vi "Get Argument Info From back Term.vi"(11 "Terminal in":refnum<vi>) -> (3 "Array":T1[](array[typedef]))   [LabVIEW 2020, in "CSM-Helper.lvclass"]
uses:
  CSM-Helper.lvclass
  Typedef/Def-Argument Info.ctl
  CSM-Helper.lvclass/CSM-Helper.ctl
  <userlib>/_NEVSTOP/Communicable State Machine(CSM)/Communicable State Machine.lvlib
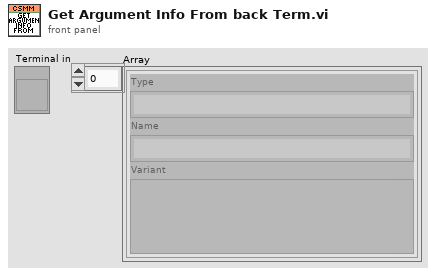
[diagram p1: front panel]
types:
  T1 = typedef "CSM-Helper.lvclass/Def-Argument Info.ctl" = cluster{"Type":string, "Name":string, "Variant":variant}
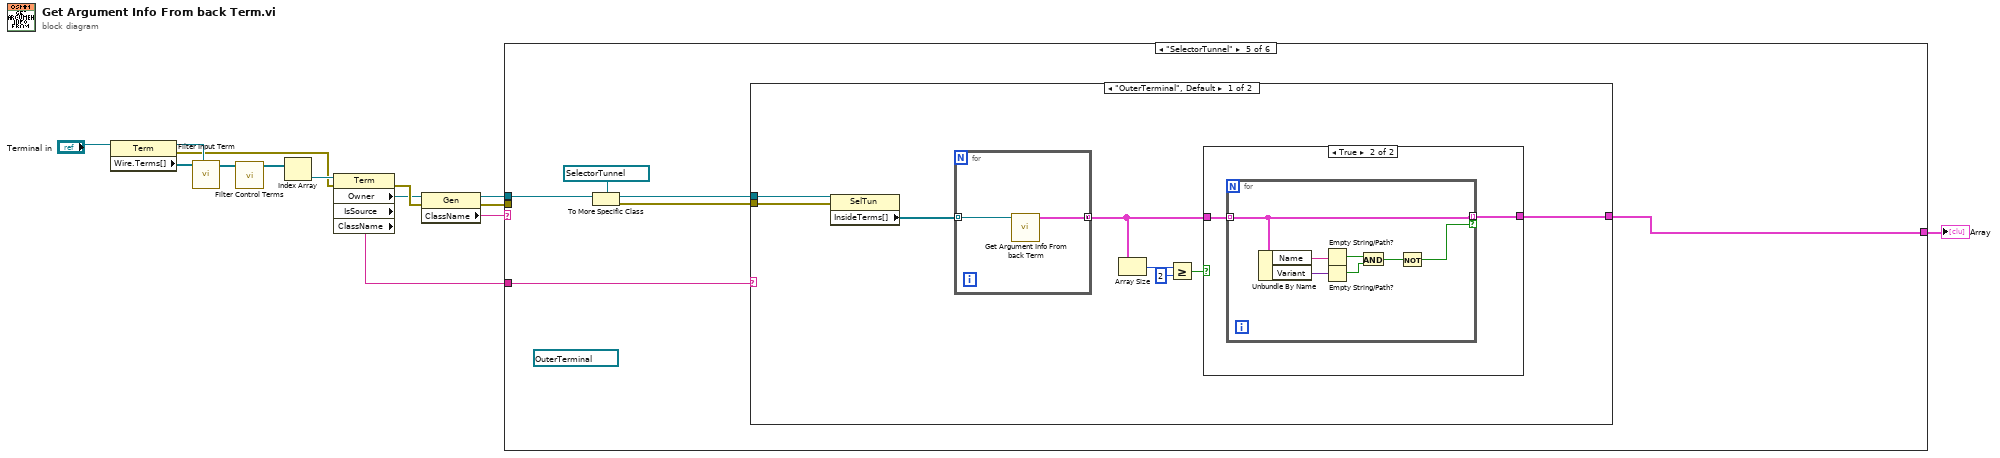
[diagram p0: block diagram]
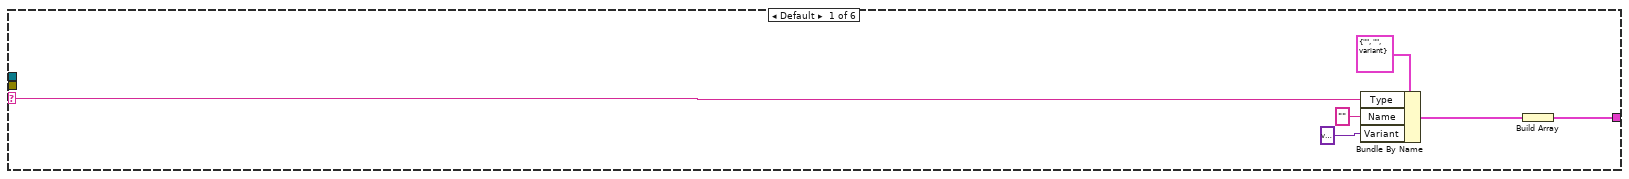
[diagram p2: hidden frame]
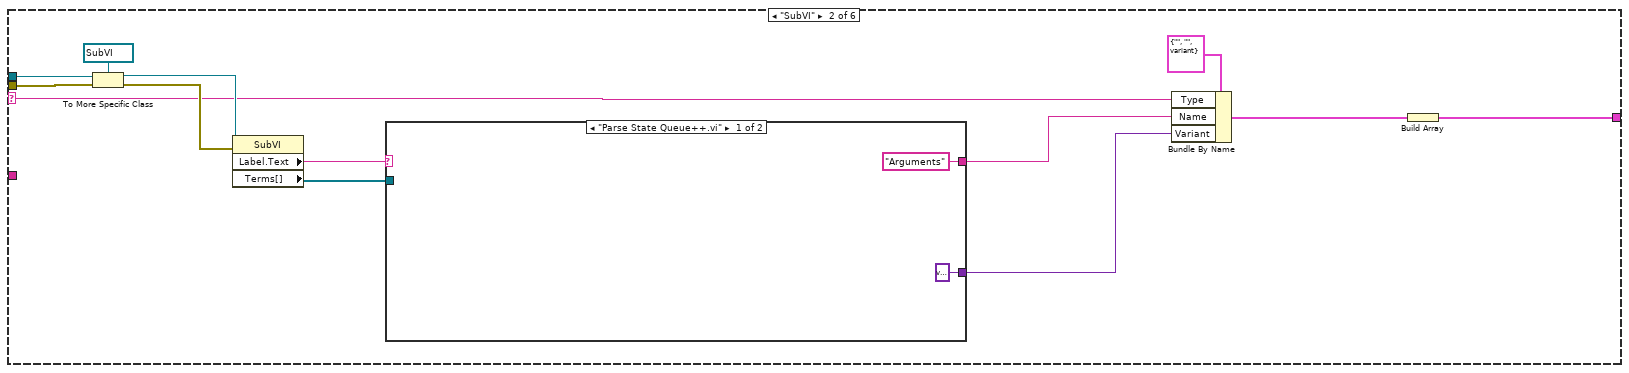
[diagram p3: hidden frame]
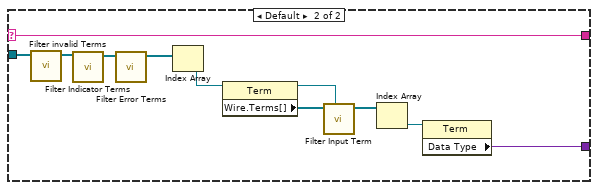
[diagram p4: hidden frame]
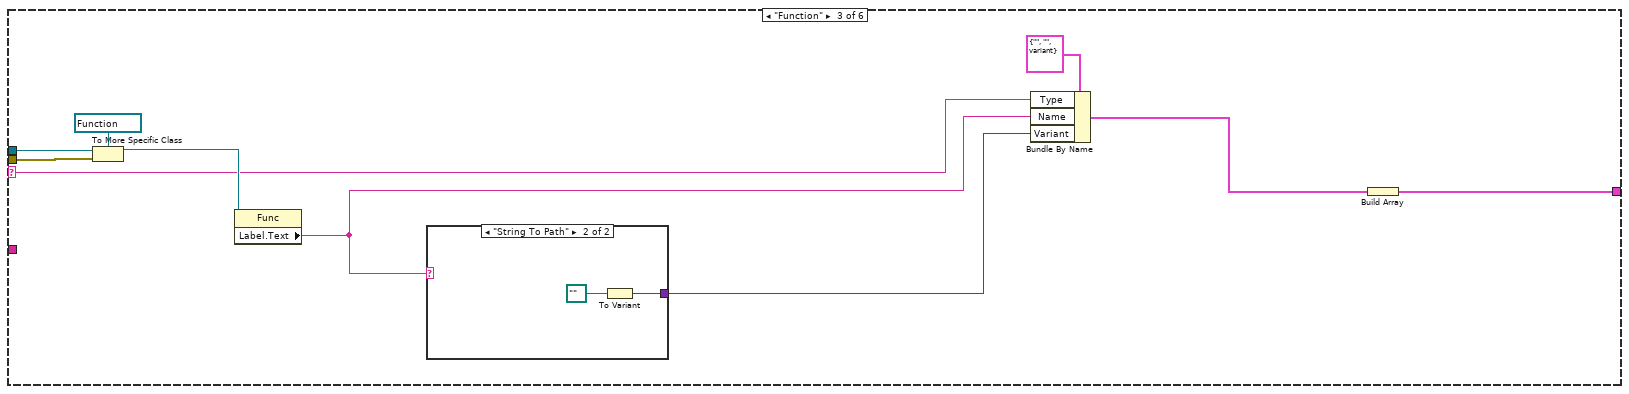
[diagram p5: hidden frame]
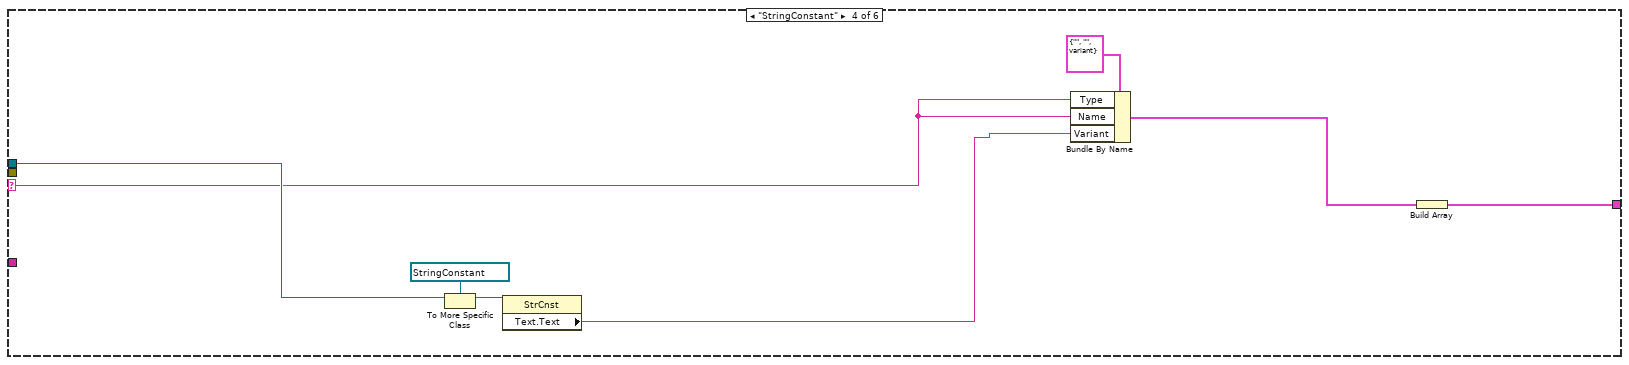
[diagram p7: hidden frame]
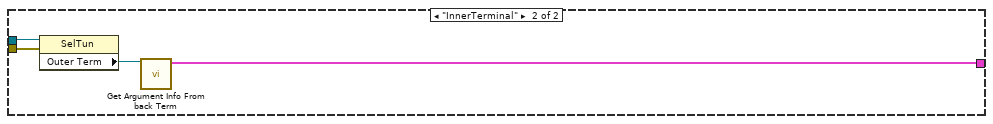
[diagram p9: hidden frame]
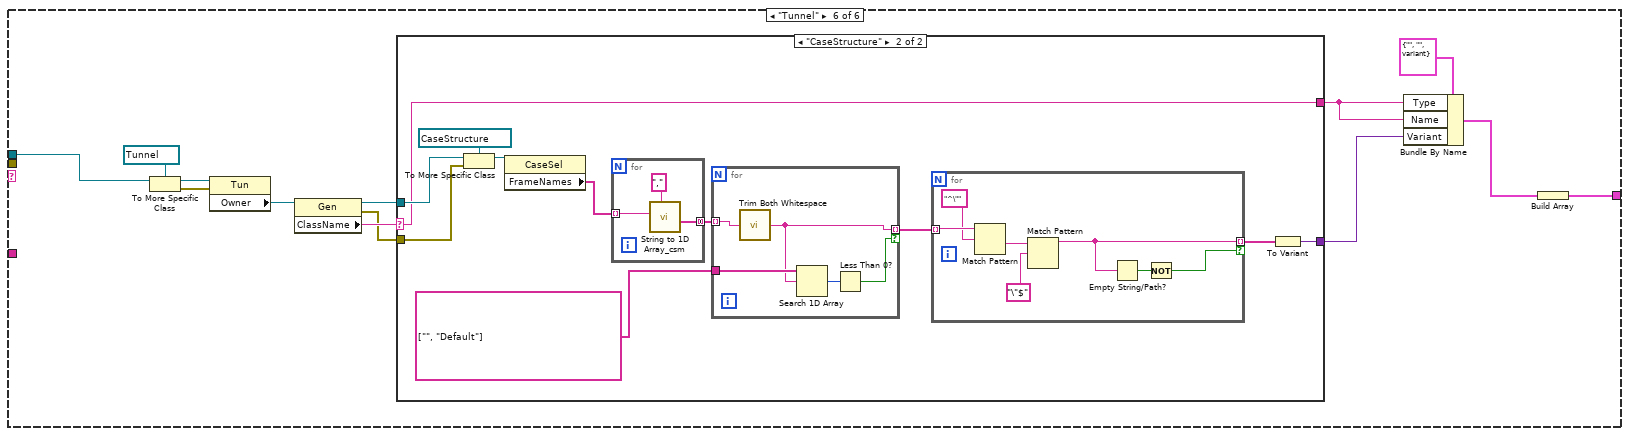
[diagram p10: hidden frame]
diagram:
  n1 = property class="Term"(reference="Terminal in") -> (reference out=w7:refnum<vi>, error out=w3:errorcluster, "Wire.Terms[]"=w8:refnum<vi>[])  [unwired: 1 in]
  n2 = call "Filter Input Term.vi"("InnerTerminal in"=w7, "Wire.Terms[] in"=w8) -> ("Wire.Terms[] out"=w6:refnum<vi>[])  [unwired: 9 in]
  n3 = call "Filter Control Terms.vi"("Terms[]"=w6) -> ("Terms[] out"=w2:refnum<vi>[])  [unwired: 10 in]
  n4 = Index Array(array=w2) -> (element=w4:refnum<vi>)  [unwired: 1 in]
  n5 = property class="Term" props=["Owner", "IsSource", "ClassName"](reference=w4, error in=w3) -> (error out=w13:errorcluster, "Owner"=w11:refnum<vi>, "ClassName"=w1:string)  [unwired: 2 out]
  n6 = property class="Gen"(reference=w11, error in=w13) -> (reference out=w12:refnum<vi>, error out=w10:errorcluster, "ClassName"=w14:string)
  n7 = case shown="\"SelectorTunnel\"" w14 {
    selector: w14 -> [w19 w26 w51 w62 _ _]
    tunnel: w12 -> [_ w31 w54 w64 w70 w109]
    tunnel: w10 -> [_ w30 w53 _ _ _]
    tunnel: [w15 w23 w47 w59 w68 w97] -> w9
    tunnel: w1 -> [_ _ _ _ w67 _]
    frame Default {
      n8 = Bundle By Name(cluster=T1 {"Type"="", "Name"="", "Variant"=variant} ("Argument"), "Type"=w19, "Name"="", "Variant"=variant) -> (w16:T1)
      n9 = Build Array(w16) -> (w15:T1[])
    }
    frame "SubVI" {
      n10 = To More Specific Class(target class=refnum<vi> refnum ("reference out"), reference=w31, error in=w30) -> (specific class reference=w32:refnum<vi>, error out=w28:errorcluster)
      n11 = property class="SubVI"(reference=w32, error in=w28) -> ("Label.Text"=w22:string, "Terms[]"=w29:refnum<vi>[])  [unwired: 2 out]
      n12 = case shown="\"Parse State Queue++.vi\"" w22 {
        selector: w22 -> [_ w36]
        tunnel: w29 -> [_ w44]
        tunnel: [variant ("Data Type") w40] -> w25
        tunnel: ["Arguments" w36] -> w21
        frame "Parse State Queue++.vi" {
        }
        frame Default {
          n13 = call "Filter invalid Terms.vi"("Terms[]"=w44) -> ("Terms[] out"=w45:refnum<vi>[])  [unwired: 10 in]
          n14 = call "Filter Indicator Terms.vi"("Terms[]"=w45) -> ("Terms[] out"=w46:refnum<vi>[])  [unwired: 10 in]
          n15 = call "Filter Error Terms.vi"("Terms[]"=w46) -> ("Terms[] out"=w43:refnum<vi>[])  [unwired: 10 in]
          n16 = Index Array(array=w43) -> (element=w42:refnum<vi>)  [unwired: 1 in]
          n17 = property class="Term"(reference=w42) -> (reference out=w38:refnum<vi>, "Wire.Terms[]"=w39:refnum<vi>[])  [unwired: 1 in, 1 out]
          n18 = call "Filter Input Term.vi"("InnerTerminal in"=w38, "Wire.Terms[] in"=w39) -> ("Wire.Terms[] out"=w37:refnum<vi>[])  [unwired: 9 in]
          n19 = Index Array(array=w37) -> (element=w41:refnum<vi>)  [unwired: 1 in]
          n20 = property class="Term"(reference=w41) -> ("Data Type"=w40:variant)  [unwired: 1 in, 2 out]
        }
      }
      n21 = Bundle By Name(cluster=T1 {"Type"="", "Name"="", "Variant"=variant} ("Argument"), "Type"=w26, "Name"=w21, "Variant"=w25) -> (w24:T1)
      n22 = Build Array(w24) -> (w23:T1[])
    }
    frame "Function" {
      n23 = To More Specific Class(target class=refnum<vi> refnum ("reference out"), reference=w54, error in=w53) -> (specific class reference=w55:refnum<vi>)  [unwired: 1 out]
      n24 = property class="Func"(reference=w55) -> ("Label.Text"=w50:string)  [unwired: 1 in, 2 out]
      n25 = case shown="\"String To Path\"" w50 {
        tunnel: [_ w57] -> w49
        frame "False", Default {
        }
        frame "String To Path" {
          n26 = To Variant(anything=path "") -> (Variant=w57:variant)
        }
      }
      n27 = Bundle By Name(cluster=T1 {"Type"="", "Name"="", "Variant"=variant} ("Argument"), "Type"=w51, "Name"=w50, "Variant"=w49) -> (w48:T1)
      n28 = Build Array(w48) -> (w47:T1[])
    }
    frame "StringConstant" {
      n29 = To More Specific Class(target class=refnum<vi> refnum ("reference out"), reference=w64) -> (specific class reference=w66:refnum<vi>)  [unwired: 1 in, 1 out]
      n30 = property class="StrCnst"(reference=w66) -> ("Text.Text"=w61:string)  [unwired: 1 in, 2 out]
      n31 = Bundle By Name(cluster=T1 {"Type"="", "Name"="", "Variant"=variant} ("Argument"), "Type"=w62, "Name"=w62, "Variant"=w61) -> (w60:T1)
      n32 = Build Array(w60) -> (w59:T1[])
    }
    frame "SelectorTunnel" {
      (unwired) refnum<vi> refnum ("reference out")
      n33 = To More Specific Class(target class=refnum<vi> refnum ("reference out"), reference=w70) -> (specific class reference=w72:refnum<vi>, error out=w69:errorcluster)  [unwired: 1 in]
      n34 = case shown="\"OuterTerminal\", Default" w67 {
        tunnel: w72 -> [w80 w96]
        tunnel: w69 -> [w78 w95]
        tunnel: [w74 w93] -> w68
        frame "OuterTerminal", Default {
          n35 = property class="SelTun"(reference=w80, error in=w78) -> ("InsideTerms[]"=w79:refnum<vi>[])  [unwired: 2 out]
          n36 = for {
            tunnel: w79 -> [w92] mode=indexing
            tunnel: [w91] -> w75 mode=concatenating
            n37 = call "Get Argument Info From back Term.vi"("Terminal in"=w92) -> ("Array"=w91:T1[])  [unwired: 10 in]
          }
          n38 = Array Size(array=w75) -> (size(s)=w77:i32)
          n39 = Greater Or Equal?(x=w77, y=2) -> (x >= y?=w73:bool)
          n40 = case shown="True" w73 {
            tunnel: w75 -> [w81 w83]
            tunnel: [w81 w82] -> w74
            frame False {
            }
            frame True {
              n41 = for {
                tunnel: w83 -> [w86] mode=indexing
                tunnel: [w86] -> w82 mode=indexing if=w84
                n42 = Unbundle By Name(w86) -> ("Name"=w90:string, "Variant"=w89:variant)
                n43 = Empty String/Path?(string/path=w90) -> (empty?=w88:bool)
                n44 = Empty String/Path?(string/path=w89) -> (empty?=w87:bool)
                n45 = And(x=w88, y=w87) -> (x .and. y?=w85:bool)
                n46 = Not(x=w85) -> (.not. x?=w84:bool)
              }
            }
          }
        }
        frame "InnerTerminal" {
          n47 = property class="SelTun"(reference=w96, error in=w95) -> ("Outer Term"=w94:refnum<vi>)  [unwired: 2 out]
          n48 = call "Get Argument Info From back Term.vi"("Terminal in"=w94) -> ("Array"=w93:T1[])  [unwired: 10 in]
        }
      }
    }
    frame "Tunnel" {
      n49 = To More Specific Class(target class=refnum<vi> refnum ("reference out"), reference=w109) -> (specific class reference=w107:refnum<vi>, error out=w106:errorcluster)  [unwired: 1 in]
      n50 = property class="Tun"(reference=w107, error in=w106) -> ("Owner"=w105:refnum<vi>)  [unwired: 2 out]
      n51 = property class="Gen"(reference=w105) -> (reference out=w103:refnum<vi>, error out=w102:errorcluster, "ClassName"=w104:string)  [unwired: 1 in]
      n52 = case shown="\"CaseStructure\"" w104 {
        selector: w104 -> [w110 w114]
        tunnel: [_ w117] -> w99
        tunnel: w103 -> [_ w116]
        tunnel: w102 -> [_ w115]
        tunnel: [w110 w114] -> w100
        frame Default {
        }
        frame "CaseStructure" {
          n53 = To More Specific Class(target class=refnum<vi> refnum ("reference out"), reference=w116, error in=w115) -> (specific class reference=w121:refnum<vi>)  [unwired: 1 out]
          n54 = property class="CaseSel"(reference=w121) -> ("FrameNames"=w118:string[])  [unwired: 1 in, 2 out]
          n55 = for {
            tunnel: [w128] -> w119 mode=concatenating
            tunnel: w118 -> [w127] mode=indexing
            n56 = call <userlib>:"String to 1D Array_csm.vi"("delimiter (Tab)"=",", "string"=w127) -> ("Array of Strings"=w128:string[])  [unwired: 9 in]
          }
          n57 = for {
            tunnel: [w124] -> w111 mode=indexing if=w122
            tunnel: w119 -> [w126] mode=indexing
            tunnel: string[] ["", "Default"] ("items to filter") -> [w125]
            n58 = call <userlib>:"Trim Both Whitespace.vi"("string"=w126) -> ("trimmed string"=w124:string)  [unwired: 1 in]
            n59 = Search 1D Array(1D array=w125, element=w124) -> (index of element=w123:i32)  [unwired: 1 in]
            n60 = Less Than 0?(x=w123) -> (x < 0?=w122:bool)
          }
          n61 = for {
            tunnel: w111 -> [w136] mode=indexing
            tunnel: [w132] -> w113 mode=indexing if=w131
            n62 = Match Pattern(string=w136, regular expression="^\"") -> (after substring=w134:string)  [unwired: 1 in, 3 out]
            n63 = Match Pattern(string=w134, regular expression="\"$") -> (before substring=w132:string)  [unwired: 1 in, 3 out]
            n64 = Empty String/Path?(string/path=w132) -> (empty?=w130:bool)
            n65 = Not(x=w130) -> (.not. x?=w131:bool)
          }
          n66 = To Variant(anything=w113) -> (Variant=w117:variant)
        }
      }
      n67 = Bundle By Name(cluster=T1 {"Type"="", "Name"="", "Variant"=variant} ("Argument"), "Type"=w100, "Name"=w100, "Variant"=w99) -> (w98:T1)
      n68 = Build Array(w98) -> (w97:T1[])
    }
  }
  "Array" <- w9
